vi "Set Event API.vi"(8 "error in (no error)":errorcluster, 10 "EventAPI":refnum<class "EventAPI.lvclass">, 11 "VolatusAPI in":refnum<class "VolatusAPI.lvclass">) -> (0 "error out":errorcluster, 3 "VolatusAPI out":refnum<class "VolatusAPI.lvclass">)   [LabVIEW 2020, in "Volatus.lvlib" / "VolatusAPI.lvclass"]
uses:
  VolatusAPI.lvclass
  VolatusAPI.lvclass/VolatusAPI.ctl
  Event API/EventAPI.lvclass
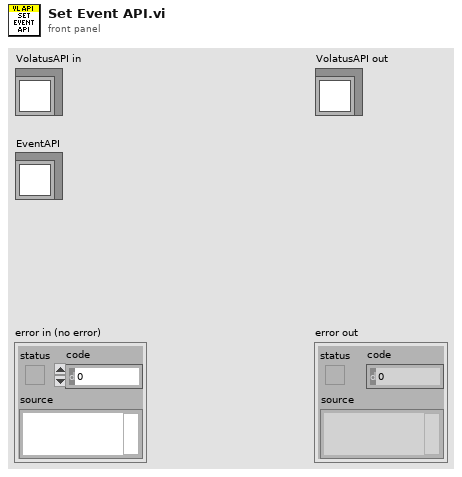
[diagram p1: front panel]
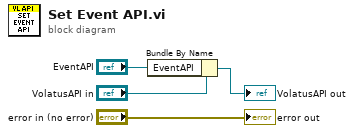
[diagram p0: block diagram]
diagram:
  n1 = Bundle By Name(cluster="VolatusAPI in", "EventAPI"="EventAPI") -> (→"VolatusAPI out":refnum<class "VolatusAPI.lvclass">)
  "error out" <- "error in (no error)"
